vi "tearDown.vi"(8 "error in (no error)":errorcluster, 11 "reference in":refnum<class "CAN Outgoing Tests.lvclass">) -> (0 "error out":errorcluster, 3 "reference out":refnum<class "CAN Outgoing Tests.lvclass">)   [LabVIEW 2017, in "CAN Outgoing Tests.lvclass"]
doc: "tearDown runs after the test method has completed. Use this method to clean up any operations or references that were opened by setUp or the test method. Unit tests should be independent of other unit tests so this VI should ensure that the next test can run in a 'clean' test environment."
uses:
  CAN Outgoing Tests.lvclass
  CAN Outgoing Tests.lvclass/CAN Outgoing Tests.ctl
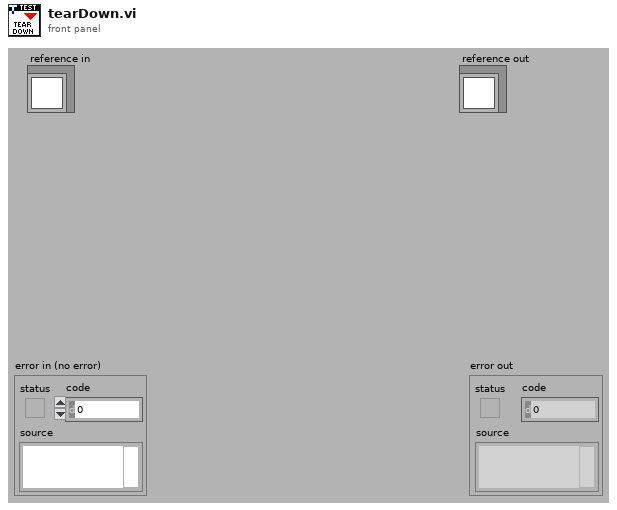
[diagram p1: front panel]
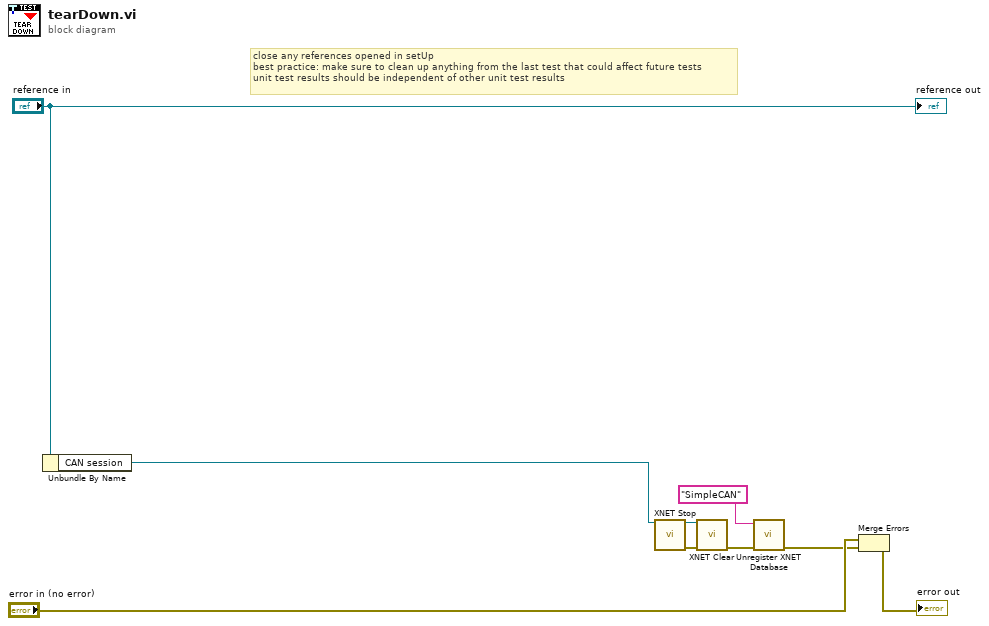
[diagram p0: block diagram]
diagram:
  # "close any references opened in setUp\nbest practice: make sure to clean up anything from the last test that could affect future tests\nunit test results should be independent of other unit test results"
  n1 = Unbundle By Name("reference in") -> ("CAN session"=w4:refnum<k21>)
  n2 = call <vilib>:"XNET Stop.vi"("session in"=w4) -> ("session out"=w6:refnum<k21>, "error out"=w5:errorcluster)  [unwired: 13 in]
  n3 = call <vilib>:"XNET Clear.vi"("session in"=w6, "error in (no error)"=w5) -> ("error out"=w3:errorcluster)  [unwired: 13 in]
  n4 = call "Unregister XNET Database.vi"("error in (no error)"=w3, "alias"="SimpleCAN") -> ("error out"=w2:errorcluster)  [unwired: 9 in]
  n5 = Merge Errors("error in (no error)", w2) -> (→"error out":errorcluster)
  "reference out" <- "reference in"
